vi "Search Packages by String.vi"() -> ()   [LabVIEW 2020]
uses:
  API Server.ctl
  Package/Get Name.vi
  Package/Get Icon.vi
  GCentral-API.lvlib
  GCentral API/GCentral API.lvclass
  Package/Package.lvclass
panel:
  in  "Search String":string
  out "Array":T1(array[cluster])
  out "error out":errorcluster
  in  "API Server":T2=enum."test"
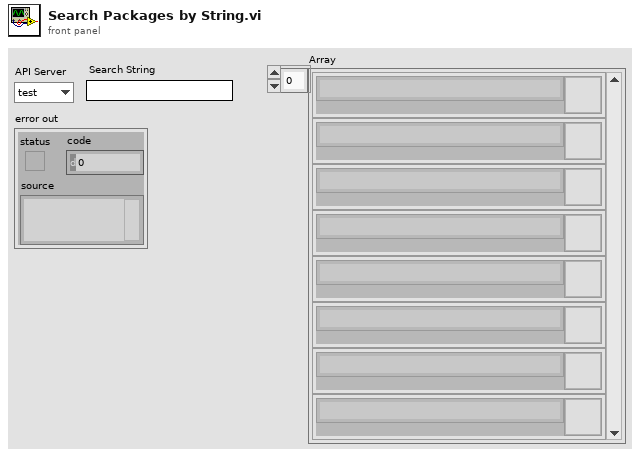
[diagram p1: front panel]
types:
  T1 = cluster{"Properties:Name":string, "Properties:Icon":picture}[]
  T2 = typedef "GCentral-API.lvlib/API Server.ctl" = enum16{"auto", "live", "test", "local"}
  T3 = cluster{"Properties:Name":string, "Properties:Icon":picture}
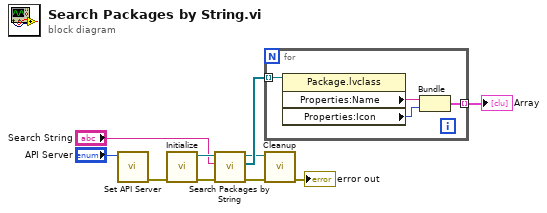
[diagram p0: block diagram]
diagram:
  n1 = call "Set API Server.vi"("API Server"="API Server") -> ("error out"=w8:errorcluster)  [unwired: 10 in]
  n2 = call "Initialize.vi"("error in (no error)"=w8) -> ("error out"=w6:errorcluster, "GCentral API out"=w5:refnum<class "GCentral API.lvclass">)  [unwired: 9 in]
  n3 = call "Search Packages by String.vi"("error in (no error)"=w6, "Search String"="Search String", "GCentral API in"=w5) -> ("error out"=w2:errorcluster, "Packages"=w4:refnum<class "Package.lvclass">[], "GCentral API out"=w3:refnum<class "GCentral API.lvclass">)  [unwired: 5 in, 1 out]
  n4 = for {
    tunnel: w4 -> [w14] mode=indexing
    tunnel: [w11] -> w7 mode=indexing
    n5 = property class="Package.lvclass"(reference=w14) -> ("Properties:Name"=w13:string, "Properties:Icon"=w12:picture)  [unwired: 1 in, 2 out]
    n6 = Bundle("Properties:Name"=w13, "Properties:Icon"=w12) -> (w11:T3)  [unwired: 1 in]
  }
  "Array" <- w7
  n7 = call "Cleanup.vi"("error in (no error)"=w2, "GCentral API in"=w3) -> ("error out"=→"error out":errorcluster)  [unwired: 9 in]
